vi "DistanceFormula.vi"(10 "Real World Coordinates":cluster{"X":sgl, "Y":sgl}, 11 "Real World Coordinates 2":cluster{"X":sgl, "Y":sgl}) -> (3 "Array":sgl[](array[numeric]))   [LabVIEW 2014]
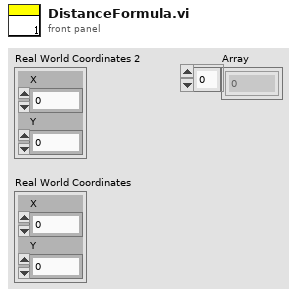
[diagram p1: front panel]
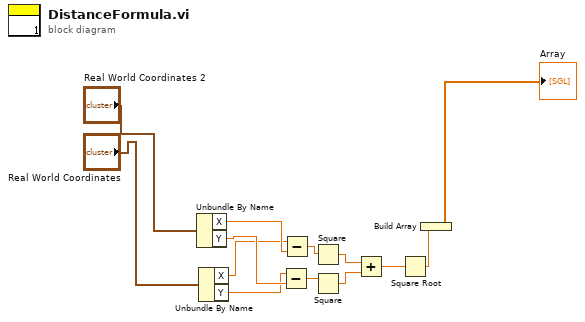
[diagram p0: block diagram]
diagram:
  n1 = Unbundle By Name("Real World Coordinates 2") -> ("X"=w4:sgl, "Y"=w6:sgl)
  n2 = Unbundle By Name("Real World Coordinates") -> ("X"=w3:sgl, "Y"=w5:sgl)
  n3 = Subtract(x=w5, y=w6) -> (x-y=w8:sgl)
  n4 = Subtract(x=w3, y=w4) -> (x-y=w7:sgl)
  n5 = Square(x=w7) -> (x^2=w9:sgl)
  n6 = Square(x=w8) -> (x^2=w10:sgl)
  n7 = Add(x=w9, y=w10) -> (x+y=w11:sgl)
  n8 = Square Root(x=w11) -> (sqrt(x)=w12:sgl)
  n9 = Build Array(w12) -> (→"Array":sgl[])
